vi "Node - Close.vi"(8 "error in (no error)":errorcluster, 11 "Node Data In":T1) -> (0 "error out":errorcluster)   [LabVIEW 2016, in "PXImc Custom Device Engine.lvlib" / "PXImc Router.lvlib"]
uses:
  PXImc Router.lvlib
  Controls/Node Data.ctl
  Controls/Table Index-Size.ctl
  <vilib>/pximc/nipximc.lvlib
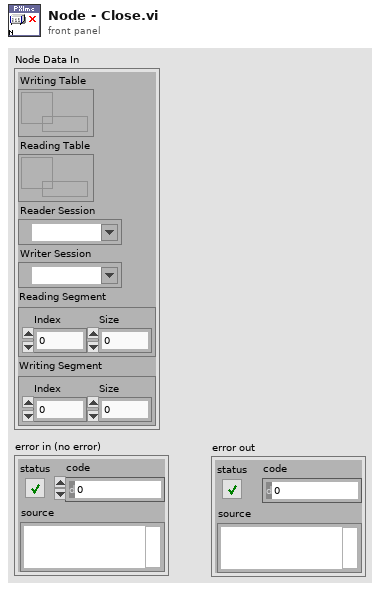
[diagram p1: front panel]
types:
  T1 = typedef "PXImc Custom Device Engine.lvlib/PXImc Router.lvlib/Node Data.ctl" = cluster{"Writing Table":refnum<data-value>, "Reading Table":refnum<data-value>, "Reader Session":refnum<k21>, "Writer Session":refnum<k21>, "Reading Segment":T2, "Writing Segment":T2}
  T2 = typedef "PXImc Custom Device Engine.lvlib/PXImc Router.lvlib/Table Index-Size.ctl" = cluster{"Index":u32, "Size":u32}
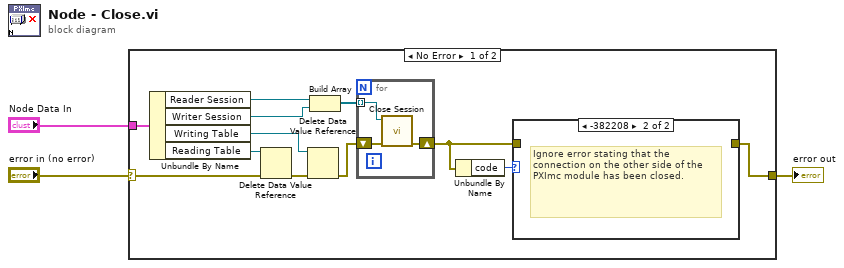
[diagram p0: block diagram]
diagram:
  n1 = case shown="No Error" "error in (no error)" {
    selector: "error in (no error)" -> [w5 w20]
    tunnel: [w11 w20] -> w3
    tunnel: "Node Data In" -> [w8 _]
    frame No Error {
      n2 = Unbundle By Name(w8) -> ("Reader Session"=w10:refnum<k21>, "Writer Session"=w9:refnum<k21>, "Writing Table"=w7:refnum<data-value>, "Reading Table"=w6:refnum<data-value>)
      n3 = Delete Data Value Reference(data value reference=w6, error in=w5) -> (error out=w4:errorcluster)  [unwired: 1 out]
      n4 = Delete Data Value Reference(data value reference=w7, error in=w4) -> (error out=w15:errorcluster)  [unwired: 1 out]
      n5 = Build Array(w10, w9) -> (w13:refnum<k21>[])
      n6 = for {
        tunnel: w13 -> [w18] mode=indexing
        shift-right: [w16] -> w14
        shift-left: w15 -> [w17]
        n7 = call <vilib>:"Close Session.vi"("error in (no error)"=w17, "session in"=w18) -> ("error out"=w16:errorcluster)  [unwired: 9 in]
      }
      n8 = Unbundle By Name(w14) -> ("code"=w12:i32)
      n9 = case shown="-382208" w12 {
        tunnel: w14 -> [w19 _]
        tunnel: [w19 _] -> w11
        frame 0, Default {
        }
        frame -382208 {
          # "Ignore error stating that the connection on the other side of the PXImc module has been closed."
        }
      }
    }
    frame Error {
    }
  }
  "error out" <- w3
